vi "MoveVelocity.vi"(3 "node":string, 4 "error in":errorcluster) -> (0 "error out":errorcluster)   [LabVIEW 2013]
uses:
  ROS/Code/SubVIs/BaxterArmsSmall.ctl
  ROS/Code/SubVIs/BaxterSide.ctl
panel:
  in  "Side":T1=enum."right"
  in  "Arm Velocities":T2
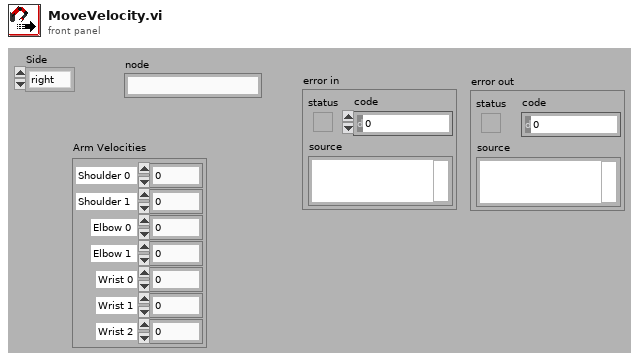
[diagram p1: front panel]
types:
  T1 = typedef "BaxterSide.ctl" = enum16{"left", "right"}
  T2 = typedef "BaxterArmsSmall.ctl" = cluster{"Elbow 0":dbl, "Elbow 1":dbl, "Shoulder 0":dbl, "Shoulder 1":dbl, "Wrist 0":dbl, "Wrist 1":dbl, "Wrist 2":dbl}
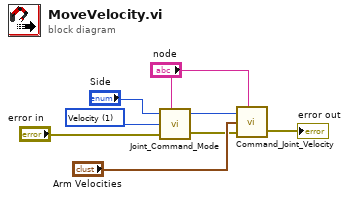
[diagram p0: block diagram]
diagram:
  w4 = u8 1 items=["Position", "Velocity", "Effort"] ("Mode")
  n1 = call "Joint_Command_Mode.vi"("Side"="Side", "node"="node", "Mode"=w4, "error in"="error in") -> ("error out"=w3:errorcluster)  [unwired: 2 in]
  n2 = call "Command_Joint_Velocity.vi"("Side"="Side", "node"="node", "Arm Velocities"="Arm Velocities", "error in"=w3) -> ("error out"=→"error out":errorcluster)  [unwired: 2 in]
